vi "Set Program State.vi"(8 "error in (no error)":errorcluster, 10 "Program Prameter":T3, 11 "ARS-0220 in":refnum<class "ARS-0220.lvclass">) -> (0 "error out":errorcluster, 2 "Status":cluster{"ACK":bool, "Error":bool, "NACK":bool}, 3 "ARS-0220 out":refnum<class "ARS-0220.lvclass">)   [LabVIEW 2021, in "Environment Chamber.lvlib" / "ARS-0220.lvclass"]
uses:
  ARS-0220.lvclass
  Support Libraries/Climatic Chamber/Private/Type Defs/Program CtrlState Enum.ctl
  Support Libraries/Climatic Chamber/Private/Type Defs/Program CtrlEndCond Enum.ctl
  ARS-0220.lvclass/ARS-0220.ctl
  Support Libraries/Climatic Chamber/Climatic Chamber.lvlib
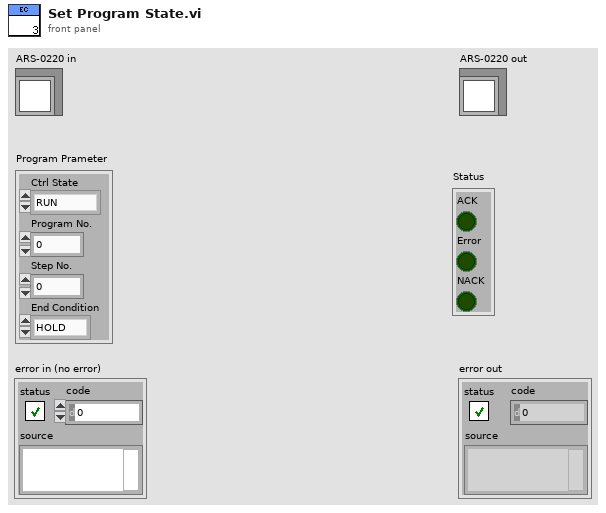
[diagram p1: front panel]
types:
  T1 = typedef "Environment Chamber.lvlib/Climatic Chamber.lvlib/Program CtrlState Enum.ctl" = enum16{"RUN", "PAUSE", "CONTINUE", "ADVANCE", "END"}
  T2 = typedef "Environment Chamber.lvlib/Climatic Chamber.lvlib/Program CtrlEndCond Enum.ctl" = enum16{"HOLD", "CONST", "OFF", "STANDBY"}
  T3 = cluster{"Ctrl State":T1, "Program No.":i32, "Step No.":i32, "End Condition":T2}
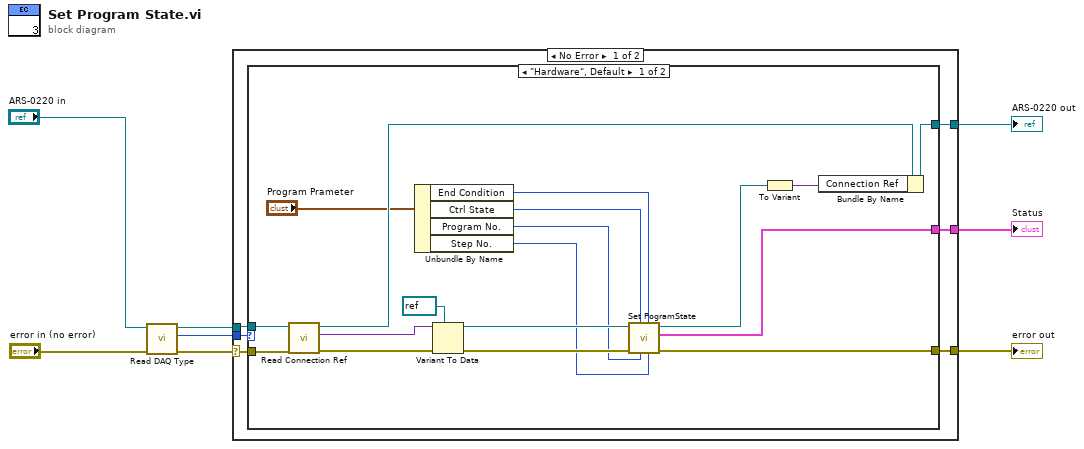
[diagram p0: block diagram]
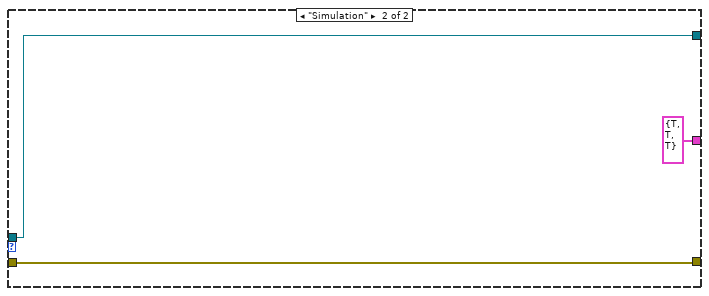
[diagram p2: hidden frame]
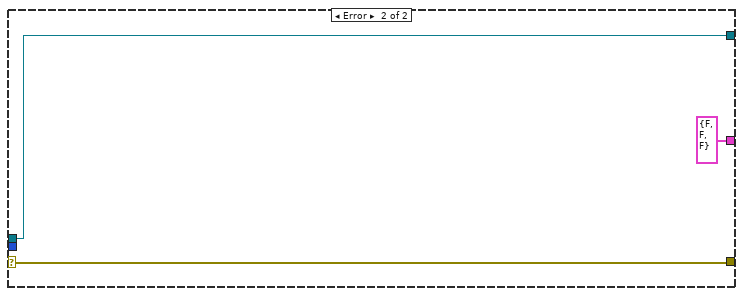
[diagram p3: hidden frame]
diagram:
  n1 = call "Read DAQ Type.vi"("error in (no error)"="error in (no error)", "ARS-0220 in"="ARS-0220 in") -> ("error out"=w7:errorcluster, "DAQ Type"=w5:enum16{"Hardware", "Simulation"}, "ARS-0220 out"=w4:refnum<class "ARS-0220.lvclass">)  [unwired: 7 in]
  n2 = case shown="No Error" w7 {
    selector: w7 -> [w12 w37]
    tunnel: w5 -> [w14 _]
    tunnel: w4 -> [w13 w38]
    tunnel: [w11 w38] -> w3
    tunnel: [w10 cluster{"ACK":bool, "Error":bool, "NACK":bool} {"ACK"=FALSE, "Error"=FALSE, "NACK"=FALSE} ("Status")] -> w2
    tunnel: [w9 w37] -> w1
    frame No Error {
      n3 = case shown="\"Hardware\", Default" w14 {
        tunnel: w13 -> [w32 w35]
        tunnel: w12 -> [w31 w34]
        tunnel: [w17 w35] -> w11
        tunnel: [w19 cluster{"ACK":bool, "Error":bool, "NACK":bool} {"ACK"=TRUE, "Error"=TRUE, "NACK"=TRUE} ("Status")] -> w10
        tunnel: [w18 w34] -> w9
        frame "Hardware", Default {
          n4 = call "Read Connection Ref.vi"("error in (no error)"=w31, "ARS-0220 in"=w32) -> ("error out"=w30:errorcluster, "Connection Ref"=w27:variant, "ARS-0220 out"=w26:refnum<class "ARS-0220.lvclass">)  [unwired: 7 in]
          n5 = Unbundle By Name("Program Prameter") -> ("End Condition"=w23:T2, "Ctrl State"=w24:T1, "Program No."=w21:i32, "Step No."=w20:i32)
          n6 = Variant To Data(error in=w30, type=refnum<visa-resource-name> refnum ("VISA resource name"), Variant=w27) -> (data=w22:refnum<visa-resource-name>, error out=w29:errorcluster)
          n7 = call "Set PogramState.vi"("Step No."=w20, "End Condition"=w23, "Program No."=w21, "Ctrl State"=w24, "error in (no error)"=w29, "VISA resource name"=w22) -> ("error out"=w18:errorcluster, "Status"=w19:cluster{"ACK":bool, "Error":bool, "NACK":bool}, "VISA resource name out"=w15:refnum<visa-resource-name>)  [unwired: 3 in]
          n8 = To Variant(anything=w15) -> (Variant=w16:variant)
          n9 = Bundle By Name(cluster=w26, "Connection Ref"=w16) -> (w17:refnum<class "ARS-0220.lvclass">)
        }
        frame "Simulation" {
        }
      }
    }
    frame Error {
    }
  }
  "error out" <- w1
  "ARS-0220 out" <- w3
  "Status" <- w2
